vi "Configure Trace Track Mode.vi"(6 "Reference Frequency (0)":dbl, 7 "Trace (1)":i32=1, 8 "error in (no error)":errorcluster, 9 "Track Mode (0: Off)":i32(ring) items=["Off", "Peak", "Frequency"], 10 "Active Channel (1)":i32=1, 11 "VISA resource name":refnum<visa-resource-name>) -> (0 "error out":errorcluster, 3 "VISA resource name out":refnum<visa-resource-name>)   [LabVIEW 2018, in "Agilent ENA Series.lvlib"]
doc: "Configures the track mode.\n\n<B>Note:</B>\nThis VI is only valid for E5060A, E5061A, E5061B."
uses:
  Agilent ENA Series.lvlib
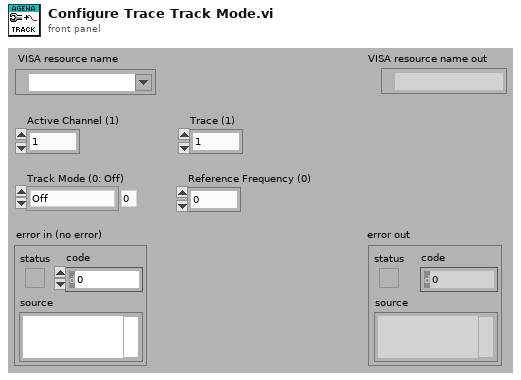
[diagram p1: front panel]
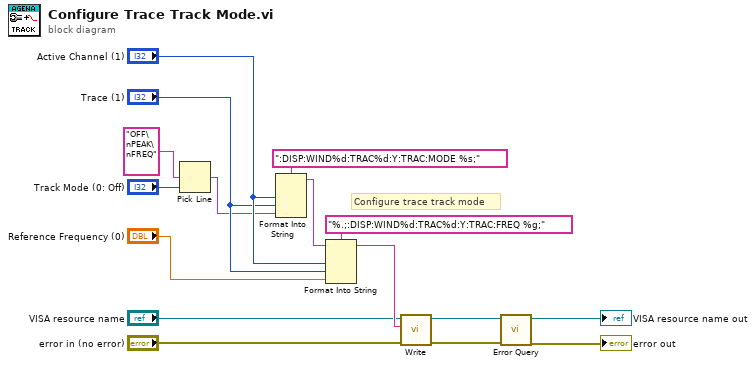
[diagram p0: block diagram]
diagram:
  # "Configure trace track mode"
  n1 = Pick Line(multi-line string="OFF\nPEAK\nFREQ", line index="Track Mode (0: Off)") -> (output string=w11:string)  [unwired: 1 out]
  n2 = Format Into String(format string=":DISP:WIND%d:TRAC%d:Y:TRAC:MODE %s;", "Active Channel (1)", "Trace (1)", w11) -> (resulting string=w10:string)  [unwired: 2 in, 1 out]
  n3 = Format Into String(format string="%.;:DISP:WIND%d:TRAC%d:Y:TRAC:FREQ %g;", initial string=w10, "Active Channel (1)", "Trace (1)", "Reference Frequency (0)") -> (resulting string=w8:string)  [unwired: 1 in, 1 out]
  n4 = call "Write.vi"("error in (no error)"="error in (no error)", "String ()"=w8, "VISA resource name"="VISA resource name") -> ("error out"=w4:errorcluster, "VISA resource name out"=w5:refnum<visa-resource-name>)  [unwired: 6 in, 1 out]
  n5 = call "Error Query.vi"("error in (no error)"=w4, "VISA resource name"=w5) -> ("error out"=→"error out":errorcluster, "VISA resource name out"=→"VISA resource name out":refnum<visa-resource-name>)  [unwired: 8 out]
